vi "Arduino to LabVIEW Communication.vi"() -> ()   [LabVIEW 2018]
uses:
  <vilib>/Instr/_visa.llb/VISA Configure Serial Port (Instr).vi
panel:
  out "loop time (ms)":u32
  out "Waveform Chart":T1(graph)
  out "Waveform Chart":u32(graph)
  out "iterations 2":u32
  out "poti_setting 2":i16
  out "bool 2":u8
  out "pressure 2":dbl
  out "pressure":dbl
  out "bool":u8
  out "poti_setting":i16
  out "iterations":u32
  out "read buffer data byte array":u8[](array[numeric]) format="%02x"
  out "Data String":string
  out "GEVE_Runtime_Data":T2
  in  "baud rate (9600)":u32=9600
  out "data string":string
  out "data byte array":u8[](array[numeric]) format="%02x"
  in  "U8 Input":u8(slide) scale=0.0..255.0
  out "Communication Timeout?":bool
  out "Serial Settings:Number of Bytes at Serial Port":u32
  in  "VISA resource name":refnum<visa-resource-name>="COM17"
  out "return count write":u32
  out "return count read":u32
  out "read buffer":string
  in  "Stop":bool
  out "Iterations":i32
  # "DEBUG AREA"
  # "iterations"
  # "poti"
  # "pressure"
  # "alarm"
  # "EOL"
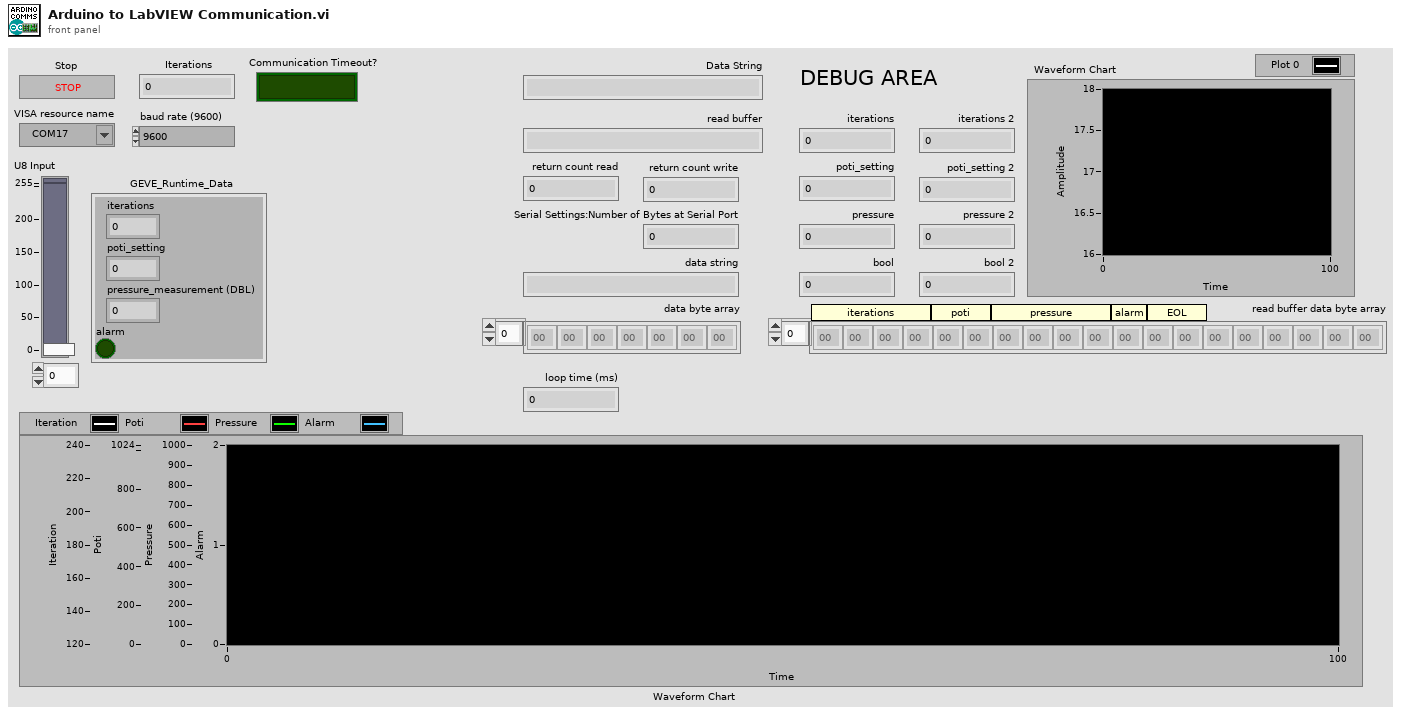
[diagram p1: front panel]
types:
  T1 = cluster{"iterations":u32, "poti_setting":i16, "pressure_measurement (DBL)":dbl, i16}
  T2 = cluster{"iterations":u32, "poti_setting":i16, "pressure_measurement (DBL)":dbl, "alarm":bool}
  T3 = enum16{"big-endian, network order", "native, host order", "little-endian"}
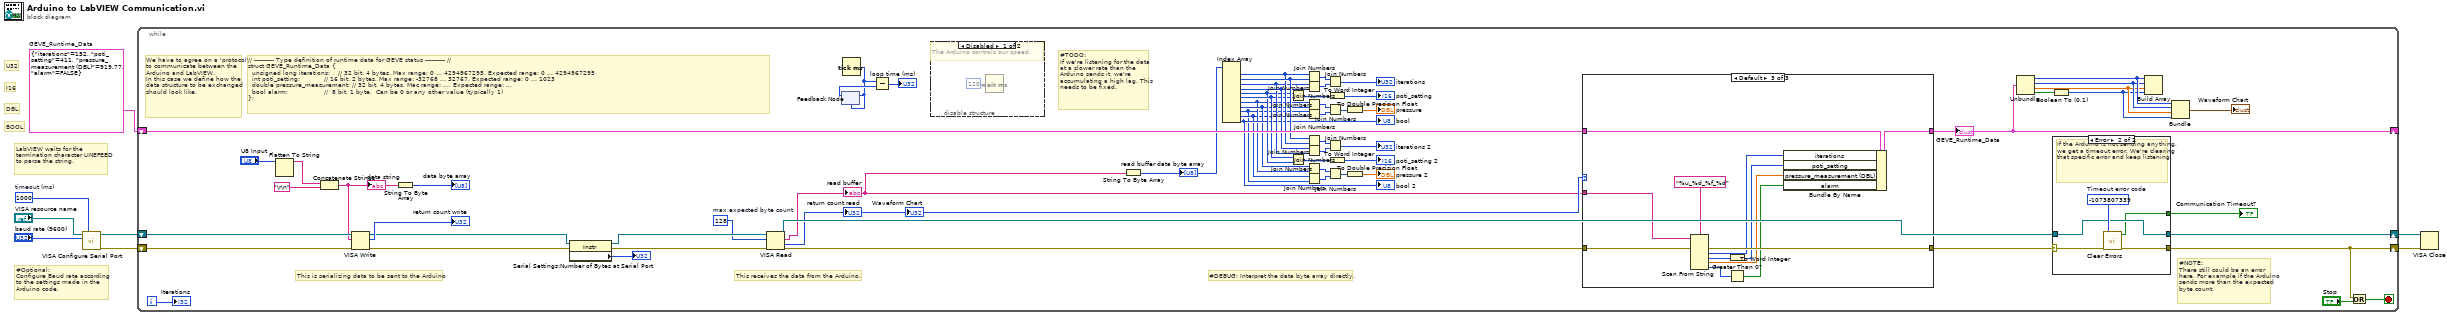
[diagram p0: block diagram]
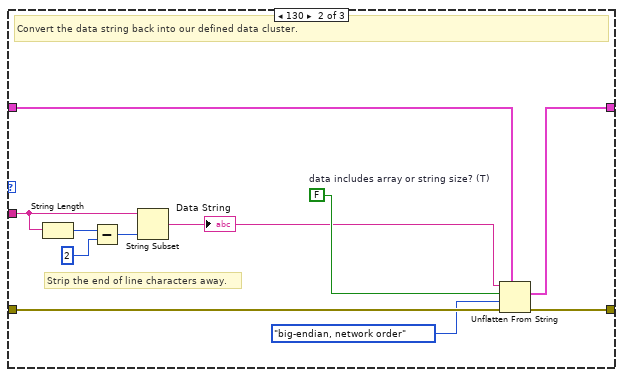
[diagram p4: hidden frame]
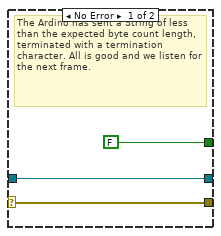
[diagram p5: hidden frame]
diagram:
  w1 = T2 {"iterations"=152, "poti_setting"=411, "pressure_measurement (DBL)"=919.77, "alarm"=FALSE}  # GEVE_Runtime_Data
  w3 = u32 1000  # timeout (ms)
  # "BOOL"
  # "DBL"
  # "I16"
  # "U32"
  # "#Optional:\nConfigure Baud rate according to the settings made in the Arduino code."
  # "LabVIEW waits for the termination character LINEFEED to parse the string."
  n1 = call-poly "VISA Configure Serial Port"("VISA resource name"="VISA resource name", "timeout (10sec)"=w3, "baud rate (9600)"="baud rate (9600)") -> ("VISA resource name out"=w8:refnum<visa-resource-name>, "error out"=w6:errorcluster)  [unwired: 11 in]
  n2 = while {
    shift-right: [w61] -> w7
    shift-left: w8 -> [w74]
    shift-right: [w62] -> w5
    shift-left: w6 -> [w73]
    shift-right: [w9] -> _
    shift-left: w1 -> [w52]
    i -> [w72]
    stop <- w69 stop-if-true
    w63 = u32 128  # max expected byte count
    # "#TODO:\nIf we're listening for the data at a slower rate than the Arduino sends it, we're accumulating a high lag. This needs to be fixed."
    # "#DEBUG: Interpret the data byte array directly."
    # "This receives the data from the Arduino."
    # "This is serializing data to be sent to the Arduino"
    # "We have to agree on a 'protocol' to communicate between the Arduino and LabVIEW.\nIn this case we define how the data structure to be exchanged should look like."
    # "// ---------- Type definition of runtime data for GEVE status ---------- //\nstruct GEVE_Runtime_Data {\n  unsigned long iterations;    // 32 bit, 4 bytes, Max range: 0 ... 4294967295, Expected range: 0 ... 4294967295\n  int poti_setting;            // 16 bit, 2 bytes, Max range: -32768 ... 32767, Expected range: 0 ... 1023\n  double pressure_measurement; // 32 bit, 4 bytes, Mac range: ..., Expected range: ...\n  bool alarm;                  //  8 bit, 1 byte,  Can be 0 or any other value (typically 1)\n};"
    # "#NOTE:\nThere still could be an error here. For example if the Arduino sends more than the expected byte count."
    n3 = Flatten To String(anything="U8 Input") -> (data string=w55:string)  [unwired: 3 in, 2 out]
    n4 = Concatenate Strings(w55, "\r\n") -> (w57:string)
    "data string" <- w57
    n5 = VISA Write(VISA resource name=w74, write buffer=w57, error in (no error)=w73) -> (VISA resource name out=w68:refnum<visa-resource-name>, return count=→"return count write":u32, error out=w67:errorcluster)
    n6 = String To Byte Array(string=w57) -> (unsigned byte array=→"data byte array":u8[])
    n7 = property class="Instr"(reference=w68, error in=w67) -> (reference out=w66:refnum<visa-resource-name>, error out=w65:errorcluster, "Serial Settings:Number of Bytes at Serial Port"=→"Serial Settings:Number of Bytes at Serial Port":u32)
    n8 = VISA Read(VISA resource name=w66, byte count=w63, error in (no error)=w65) -> (VISA resource name out=w60:refnum<visa-resource-name>, read buffer=w20:string, return count=w21:u32, error out=w19:errorcluster)
    "read buffer" <- w20
    "return count read" <- w21
    "Waveform Chart" <- w21
    n9 = Tick Count (ms)() -> (millisecond timer value=w10:u32)
    n10 = feedback-in #1(w10) -> ()
    n11 = feedback #1(w10) -> (w12:u32)
    n12 = Subtract(x=w10, y=w12) -> (x-y=→"loop time (ms)":u32)
    n13 = disable-structure shown="Disabled" {
      frame Disabled {
        # "The Arduino controls our speed."
        n14 = Wait (ms)(milliseconds to wait=u32 120) -> ()  [unwired: 1 out]
      }
      frame Enabled {
      }
    }
    n15 = String To Byte Array(string=w20) -> (unsigned byte array=w51:u8[])
    "read buffer data byte array" <- w51
    n16 = Index Array(array=w51) -> (element #1=w31:u8, element #2=w32:u8, element #3=w29:u8, element #4=w30:u8, element #5=w27:u8, element #6=w28:u8, element #7=w24:u8, element #8=w25:u8, element #9=w22:u8, element #10=w23:u8, element #11=→"bool" →"bool 2":u8)  [unwired: 11 in]
    n17 = Join Numbers(hi=w27, lo=w28) -> ((hi.lo)=w47:u16)
    n18 = Join Numbers(hi=w28, lo=w27) -> ((hi.lo)=w36:u16)
    n19 = Join Numbers(hi=w31, lo=w32) -> ((hi.lo)=w50:u16)
    n20 = Join Numbers(hi=w29, lo=w30) -> ((hi.lo)=w49:u16)
    n21 = Join Numbers(hi=w24, lo=w25) -> ((hi.lo)=w44:u16)
    n22 = Join Numbers(hi=w22, lo=w23) -> ((hi.lo)=w45:u16)
    n23 = Join Numbers(hi=w32, lo=w31) -> ((hi.lo)=w33:u16)
    n24 = Join Numbers(hi=w30, lo=w29) -> ((hi.lo)=w34:u16)
    n25 = Join Numbers(hi=w25, lo=w24) -> ((hi.lo)=w39:u16)
    n26 = Join Numbers(hi=w23, lo=w22) -> ((hi.lo)=w38:u16)
    n27 = Join Numbers(hi=w50, lo=w49) -> ((hi.lo)=→"iterations":u32)
    n28 = Join Numbers(hi=w44, lo=w45) -> ((hi.lo)=w43:u32)
    n29 = Join Numbers(hi=w33, lo=w34) -> ((hi.lo)=→"iterations 2":u32)
    n30 = Join Numbers(hi=w39, lo=w38) -> ((hi.lo)=w40:u32)
    n31 = To Word Integer(number=w47) -> (16bit integer=→"poti_setting":i16)
    n32 = To Word Integer(number=w36) -> (16bit integer=→"poti_setting 2":i16)
    n33 = To Double Precision Float(number=w43) -> (double precision float=→"pressure":dbl)
    n34 = To Double Precision Float(number=w40) -> (double precision float=→"pressure 2":dbl)
    n35 = case shown="Default" w21 {
      tunnel: w19 -> [w76 w87 w95]
      tunnel: [w76 w86 w94] -> w53
      tunnel: w52 -> [w77 w85 w100]
      tunnel: [w77 w84 w99] -> w9
      tunnel: w20 -> [_ w78 w96]
      frame 0 {
      }
      frame 130 {
        w88 = FALSE  # data includes array or string size? (T)
        # "Strip the end of line characters away."
        # "Convert the data string back into our defined data cluster."
        n36 = String Length(string=w78) -> (length=w83:i32)
        n37 = Subtract(x=w83, y=2) -> (x-y=w81:i32)
        n38 = String Subset(string=w78, length (rest)=w81) -> (substring=w80:string)  [unwired: 1 in]
        "Data String" <- w80
        n39 = Unflatten From String(type=w85, binary string=w80, data includes array or string size? (T)=w88, byte order (0:big-endian, network order)=T3."big-endian, network order", error in (no error)=w87) -> (value=w84:T2, error out=w86:errorcluster)  [unwired: 1 out]
      }
      frame Default {
        n40 = Scan From String(format string="%u_%d_%f_%d", input string=w96, error in=w95) -> (error out=w94:errorcluster, output 1=w89:u32, output 2=w98:i32, output 3=w90:dbl, output 4=w93:i32)  [unwired: 5 in, 2 out]
        n41 = To Word Integer(number=w98) -> (16bit integer=w91:i16)
        n42 = Greater Than 0?(x=w93) -> (x > 0?=w92:bool)
        n43 = Bundle By Name(cluster=w100, "iterations"=w89, "poti_setting"=w91, "pressure_measurement (DBL)"=w90, "alarm"=w92) -> (w99:T2)
      }
    }
    "GEVE_Runtime_Data" <- w9
    n44 = Unbundle(w9) -> ("iterations"=w18:u32, "poti_setting"=w17:i16, "pressure_measurement (DBL)"=w15:dbl, "alarm"=w14:bool)
    n45 = Boolean To (0,1)(Boolean=w14) -> (0, 1=w13:i16)
    n46 = case shown="Error" w53 {
      selector: w53 -> [w103 w108]
      tunnel: [w103 w106] -> w62
      tunnel: [w102 w105] -> w61
      tunnel: w60 -> [w102 w105]
      tunnel: [FALSE ("specific error cleared?") w104] -> w59
      frame No Error {
        # "The Ardino has sent a String of less than the expected byte count length, terminated with a termination character. All is good and we listen for the next frame."
      }
      frame Error {
        w107 = -1073807339  # Timeout error code
        # "If the Arduino is not sending anything, we get a timeout error. We're clearing that specific error and keep listening."
        n47 = call <vilib>:"Clear Errors.vi"("error in (no error)"=w108, "specific error code to clear (0: all)"=w107) -> ("error out"=w106:errorcluster, "specific error cleared?"=w104:bool)  [unwired: 4 in]
      }
    }
    "Communication Timeout?" <- w59
    n48 = Build Array(w18, w17, w15, w13) -> ()  [unwired: 1 out]
    n49 = Bundle("iterations"=w18, "poti_setting"=w17, "pressure_measurement (DBL)"=w15, w13) -> (→"Waveform Chart":T1)  [unwired: 1 in]
    n50 = Or(x=w62, y="Stop") -> (x .or. y?=w69:bool)
    "Iterations" <- w72
  }
  n51 = VISA Close(VISA resource name=w7, error in (no error)=w5) -> ()  [unwired: 1 out]
